vi "Unflatten from String.vi"(8 "error in (no error)":errorcluster, 10 "Flattened String":string, 11 "Message Flattener in":refnum<class "Message Flattener.lvclass">) -> (0 "error out":errorcluster, 1 "priority":i32, 2 "Message":refnum<class "Message.lvclass">, 3 "Message Flattener out":refnum<class "Message Flattener.lvclass">)   [LabVIEW 2020, in "Message Flattener.lvclass"]
doc: "This method uses the Unflatten to String function to turn a string into a message object. Override this method to implement a different serialization scheme."
uses:
  Message Flattener.lvclass
  <vilib>/ActorFramework/Message/Message.lvclass
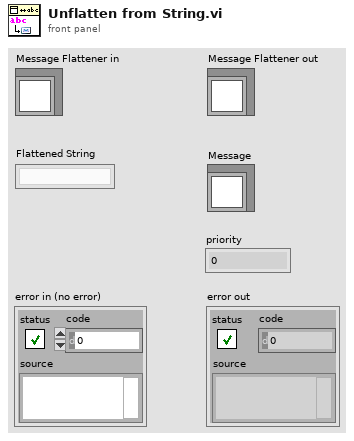
[diagram p1: front panel]
types:
  T1 = cluster{"Actor Framework:Message":refnum<class "Message.lvclass">, "priority":i32}
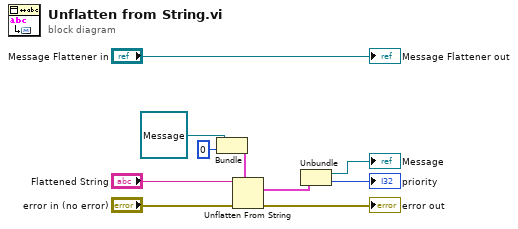
[diagram p0: block diagram]
diagram:
  n1 = Bundle("Actor Framework:Message"=refnum<class "Message.lvclass"> refnum, "priority"=0) -> (w8:T1)  [unwired: 1 in]
  n2 = Unflatten From String(type=w8, binary string="Flattened String", error in (no error)="error in (no error)") -> (value=w9:T1, error out=→"error out":errorcluster)  [unwired: 2 in, 1 out]
  n3 = Unbundle(w9) -> ("Actor Framework:Message"=→"Message":refnum<class "Message.lvclass">, "priority"=→"priority":i32)
  "Message Flattener out" <- "Message Flattener in"
